vi "ExSubNframeColMultiImageFast.vi"(2 "image handles":u32[](array[numeric]), 3 "error in (no error)":errorcluster, 4 "Number of Images":u32=1 min=1 step=1, 5 "Handle Cluster":T1) -> (0 "error out":errorcluster, 1 "Handle Cluster":T1)   [LabVIEW 2010]
panel:
  # "ExSubNframeCol:\nThis is a sub VI that collects N frames from the camera\nsystem. This assumes camera has been setup and \ninitialized and that the start camera is done. It also \nassumes the camera has circular buffer capabillities.\nThis is not true for all cameras, especially older \nPhotometrics cameras."
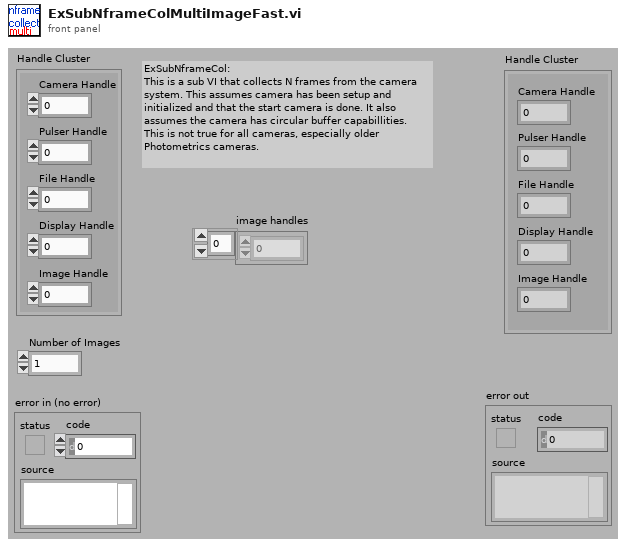
[diagram p1: front panel]
types:
  T1 = cluster{"Camera Handle":u32, "Pulser Handle":u32, "File Handle":u32, "Display Handle":u32, "Image Handle":u32}
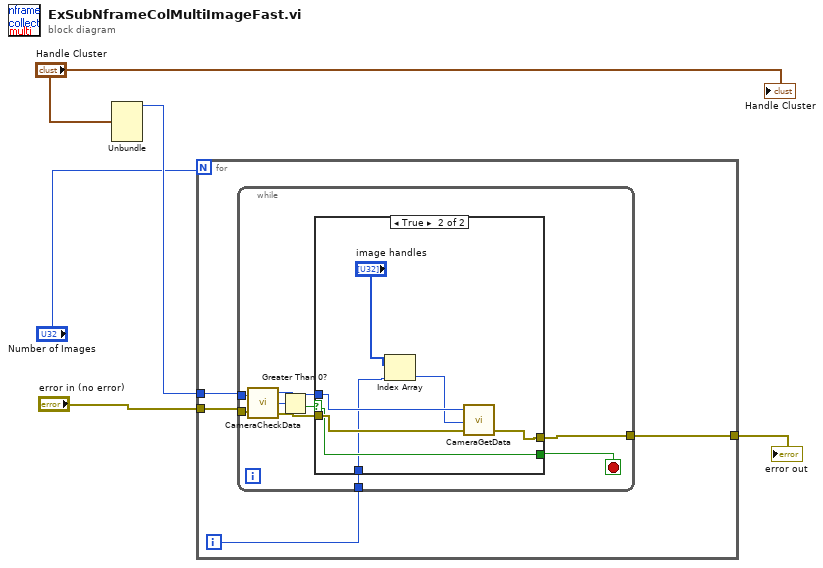
[diagram p0: block diagram]
diagram:
  n1 = Unbundle("Handle Cluster") -> ("Camera Handle"=w5:u32)  [unwired: 4 out]
  n2 = for {
    N: "Number of Images" -> [_]
    tunnel: w5 -> [w9]
    tunnel: "error in (no error)" -> [w8]
    tunnel: [w6] -> w1
    i -> [w7]
    n3 = while {
      tunnel: w8 -> [w17]
      tunnel: w9 -> [w16]
      tunnel: [w11] -> w6
      tunnel: w7 -> [w10]
      stop <- w12 stop-if-true
      n4 = call <userlib>:"CameraCheckData.vi"("Camera Handle"=w16, "error in"=w17) -> ("Camera Handle"=w14:u32, "Number Of Frames Available"=w18:i32, "error out"=w13:errorcluster)
      n5 = Greater Than 0?(x=w18) -> (x > 0?=w15:bool)
      n6 = case shown="True" w15 {
        selector: w15 -> [w19 w25]
        tunnel: w14 -> [_ w27]
        tunnel: w13 -> [w20 w26]
        tunnel: [w19 w25] -> w12
        tunnel: [w20 w24] -> w11
        tunnel: w10 -> [_ w23]
        frame False {
        }
        frame True {
          n7 = Index Array(array="image handles", index=w23) -> (element=w21:u32)
          n8 = call <userlib>:"CameraGetData.vi"("error in"=w26, "Data Handle"=w21, "Camera Handle"=w27) -> ("error out"=w24:errorcluster)  [unwired: 2 out]
        }
      }
    }
  }
  "error out" <- w1
  "Handle Cluster" <- "Handle Cluster"
